vi "TCP service test.vi"() -> ()   [LabVIEW 2014]
panel:
  out "长度":i32
  in  "发送的消息":string="当前正从客户端%s（端口%d）访问TCP Named Service - Server.vi。"
  in  "停止":bool
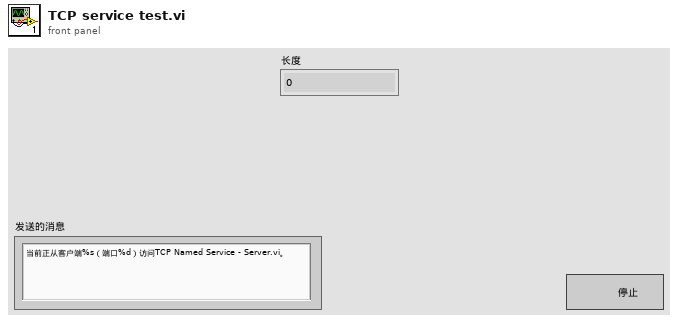
[diagram p1: front panel]
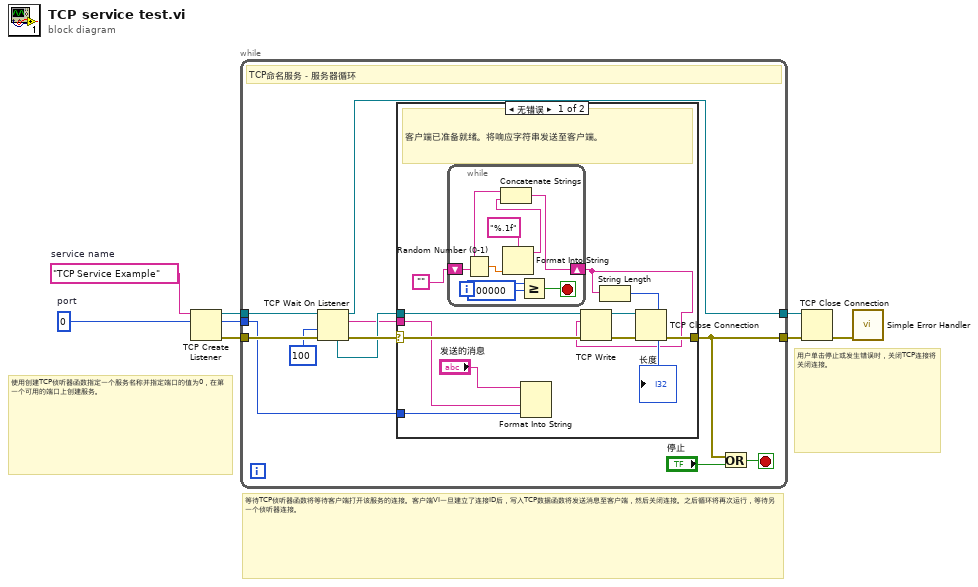
[diagram p0: block diagram]
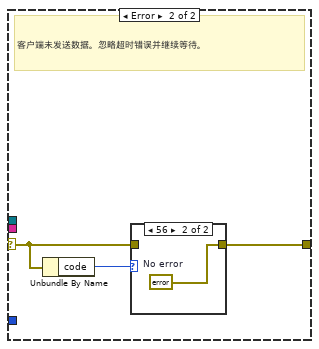
[diagram p2: hidden frame]
diagram:
  w2 = u16 0  # port
  w1 = "TCP Service Example"  # service name
  # "用户单击停止或发生错误时，关闭TCP连接将关闭连接。"
  # "等待TCP侦听器函数将等待客户端打开该服务的连接。客户端VI一旦建立了连接ID后，写入TCP数据函数将发送消息至客户端，然后关闭连接。之后循环将再次运行，等待另一个侦听器连接。"
  # "使用创建TCP侦听器函数指定一个服务名称并指定端口的值为0，在第一个可用的端口上创建服务。"
  n1 = TCP Create Listener(10:w2, 11:w1) -> (0:w7:errorcluster, 2:w4:u16, 3:w8:refnum<k5>)  [unwired: 3 in]
  n2 = while {
    tunnel: [w12] -> w5
    tunnel: w8 -> [w19]
    tunnel: w7 -> [w17]
    tunnel: [w9] -> w6
    tunnel: w4 -> [w15]
    stop <- w14 stop-if-true
    # "TCP命名服务－服务器循环"
    n3 = TCP Wait On Listener(8:w17, 9:100 ("timeout ms (25000)"), 11:w19) -> (0:w18:errorcluster, 2:w10:string, 3:w9:refnum<k5>, 4:w16:refnum<k5>)  [unwired: 1 in, 1 out]
    n4 = case shown="无错误" w18 {
      selector: w18 -> [w30 w41]
      tunnel: [w25 w39] -> w12
      tunnel: w16 -> [w26 _]
      tunnel: w15 -> [w28 _]
      tunnel: w10 -> [w27 _]
      frame No Error {
        # "客户端已准备就绪。将响应字符串发送至客户端。"
        n5 = while {
          shift-right: [w34] -> w20
          shift-left: "" -> [w35]
          i -> [w38]
          stop <- w36 stop-if-true
          n6 = Random Number (0-1)() -> (number: 0 to 1=w33:dbl)
          n7 = Format Into String(format string="%.1f" ("格式字符串"), w33) -> (resulting string=w31:string)  [unwired: 2 in, 1 out]
          n8 = Concatenate Strings(w35, w31) -> (w34:string)
          n9 = Greater Or Equal?(x=w38, y=900000) -> (x >= y?=w36:bool)
        }
        n10 = Format Into String(initial string="发送的消息", w27, w28) -> ()  [unwired: 2 in, 2 out]
        n11 = TCP Write(connection ID=w26, data in=w20, error in (no error)=w30) -> (connection ID out=w24:refnum<k5>, error out=w29:errorcluster)  [unwired: 1 in, 1 out]
        n12 = String Length(string=w20) -> (length=→"长度":i32)
        n13 = TCP Close Connection(connection ID=w24, error in (no error)=w29) -> (error out=w25:errorcluster)  [unwired: 1 in, 1 out]
      }
      frame Error {
        # "客户端未发送数据。忽略超时错误并继续等待。"
        n14 = Unbundle By Name(w41) -> ("code"=w40:i32)
        n15 = case shown="56" w40 {
          tunnel: w41 -> [w42 _]
          tunnel: [w42 w43] -> w39
          frame Default {
          }
          frame 56 {
            w43 = errorcluster {"status"=FALSE, "code"=0, "source"=""}  # No error
          }
        }
      }
    }
    n16 = Or(x=w12, y="停止") -> (x .or. y?=w14:bool)
  }
  n17 = TCP Close Connection(connection ID=w6, error in (no error)=w5) -> (error out=w3:errorcluster)  [unwired: 1 in, 1 out]
  n18 = call <vilib>:"Simple Error Handler.vi"("error in (no error)"=w3) -> ()  [unwired: 4 in, 5 out]
